vi "GenerateParComments.vi"(1 "Desciptions":string[](array[string]), 2 "Types":variant[](array[variant]), 5 "error in (no error)":errorcluster) -> (15 "DescriptionString":string, 16 "Names":string[](array[string]), 19 "error out":errorcluster)   [LabVIEW 2018, in "Python.lvclass"]
uses:
  Python.lvclass
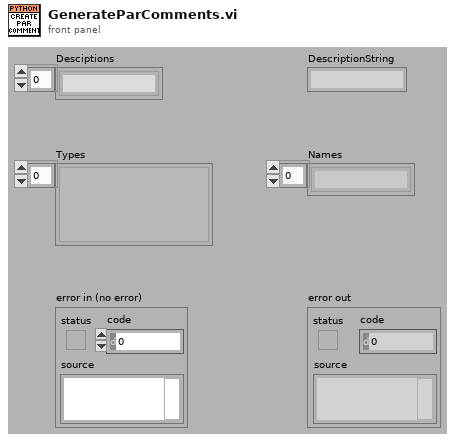
[diagram p1: front panel]
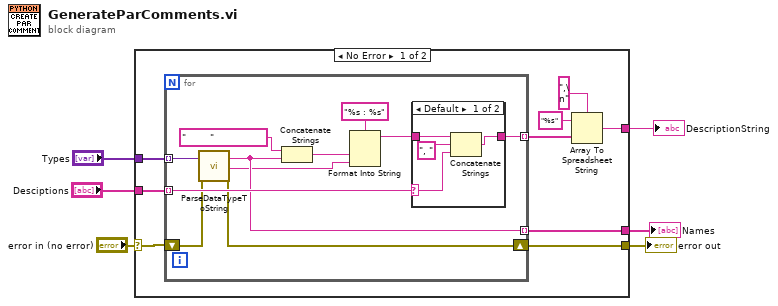
[diagram p0: block diagram]
diagram:
  n1 = case shown="No Error" "error in (no error)" {
    selector: "error in (no error)" -> [w8 w32]
    tunnel: [w7 w32] -> w5
    tunnel: "Types" -> [w13 _]
    tunnel: "Desciptions" -> [w12 _]
    tunnel: [w11 _] -> w2
    tunnel: [w9 _] -> w1
    frame No Error {
      n2 = for {
        tunnel: w13 -> [w20] mode=indexing
        tunnel: w12 -> [w23] mode=indexing
        tunnel: [w19] -> w9 mode=indexing
        tunnel: [w22] -> w10 mode=indexing
        shift-right: [w17] -> w7
        shift-left: w8 -> [w16]
        n3 = call "ParseDataTypeToString.vi"("Variant"=w20, "error in (no error)"=w16) -> ("Name"=w19:string, "String"=w18:string, "error out"=w17:errorcluster)  [unwired: 15 in]
        n4 = Concatenate Strings("        " ("string"), w19) -> (w26:string)
        n5 = Format Into String(format string="%s : %s", w26, w18) -> (resulting string=w21:string)  [unwired: 2 in, 1 out]
        n6 = case shown="Default" w23 {
          selector: w23 -> [w28 _]
          tunnel: [w27 w31] -> w22
          tunnel: w21 -> [w29 w31]
          frame Default {
            n7 = Concatenate Strings(w29, ", " ("string"), w28) -> (w27:string)
          }
          frame "" {
          }
        }
      }
      n8 = Array To Spreadsheet String(delimiter (Tab)=",\n", array=w10, 3:"%s" ("format string")) -> (spreadsheet string=w11:string)
    }
    frame Error {
    }
  }
  "error out" <- w5
  "DescriptionString" <- w2
  "Names" <- w1
